vi "TEST-runner.vi"() -> ()   [LabVIEW 2016]
uses:
  Classes/Controllers/Motion/Copy of Motion Folder/Motion.lvclass
  Classes/Controllers/Camera/Copy of Controller Folder/Controller.lvclass
panel:
  in  "loop time":i32
  in  "START":bool
  in  "stop":bool
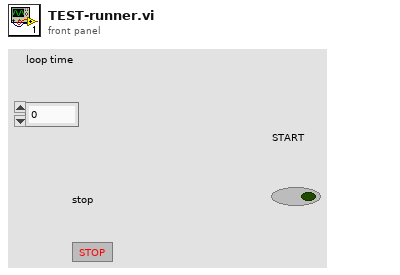
[diagram p1: front panel]
types:
  T1 = typedef "Controller.lvclass/Controllers.ctl" = cluster{"Copy of Motion.lvclass":refnum<class "Motion.lvclass">, "Copy of I-O.lvclass":refnum<class "I-O.lvclass">, "Copy of Dispenser.lvclass":refnum<class "Dispenser.lvclass">}
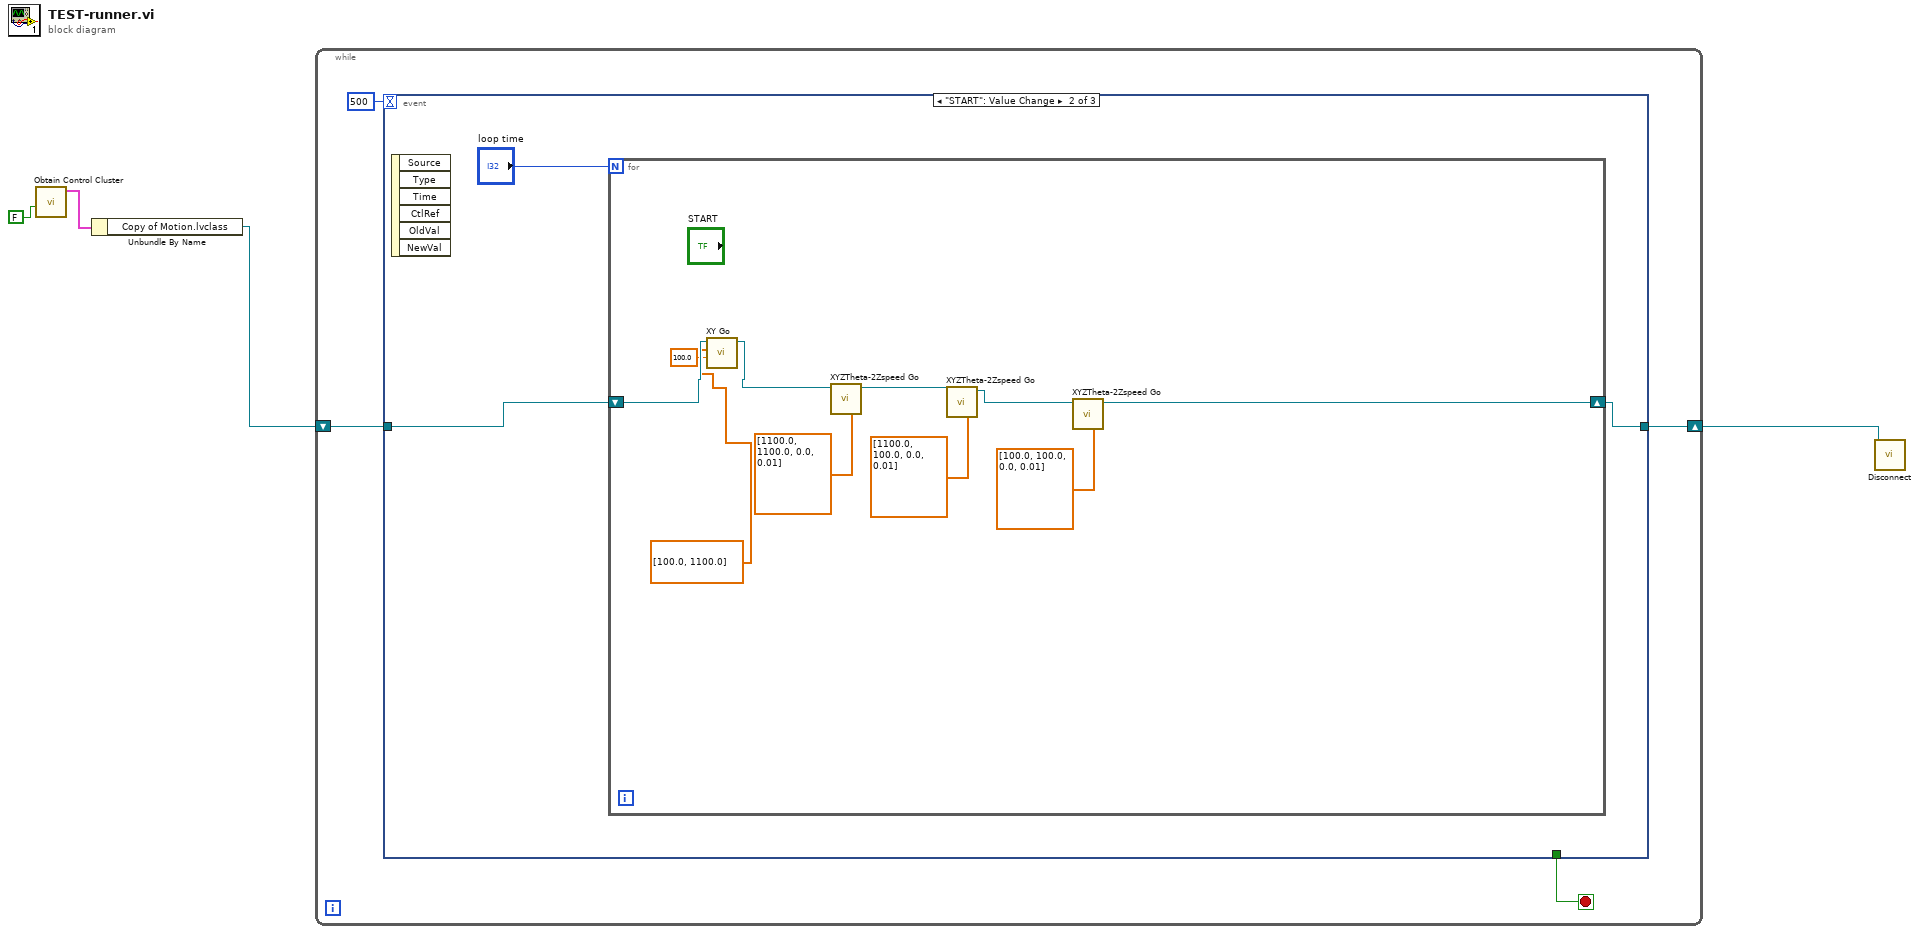
[diagram p0: block diagram]
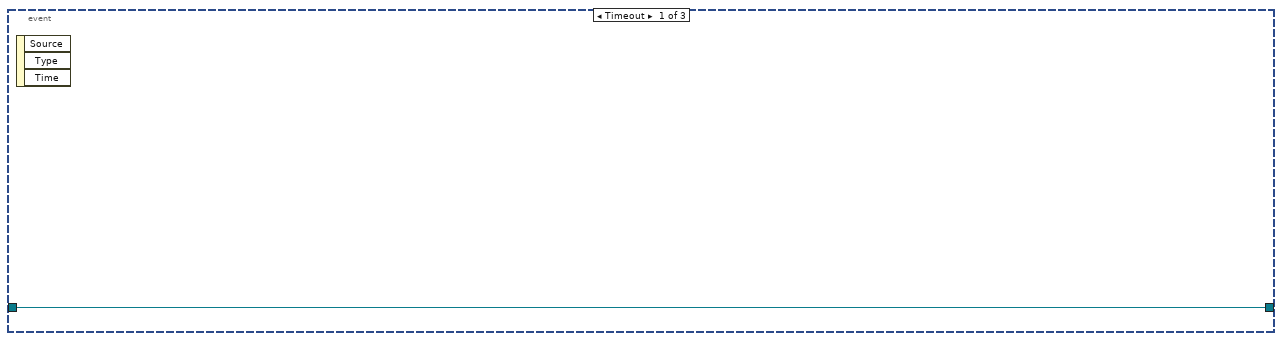
[diagram p2: hidden frame]
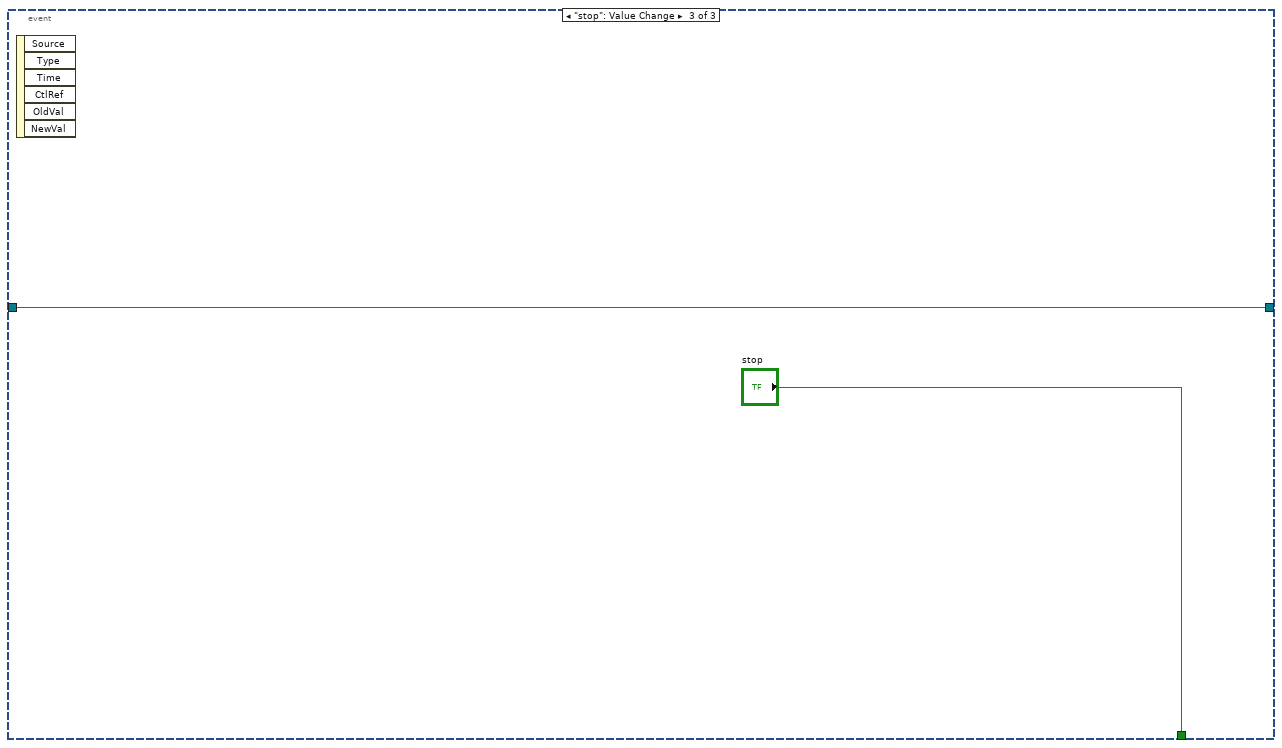
[diagram p3: hidden frame]
diagram:
  n1 = call "Obtain Control Cluster.vi"("I/O"=FALSE) -> ("Control Out"=w4:T1)  [unwired: 10 in]
  n2 = Unbundle By Name(w4) -> ("Copy of Motion.lvclass"=w2:refnum<class "Motion.lvclass">)
  n3 = while {
    shift-right: [w7] -> w1
    shift-left: w2 -> [w8]
    stop <- w5 stop-if-true
    n4 = event shown="[1] \"START\": Value Change" {
      selector: _ -> [_ _ _]
      dyn-events: _ -> [_ _ _]
      timeout: 500 -> [_ _ _]
      tunnel: w8 -> [w9 w11 w24]
      tunnel: [w9 w10 w24] -> w7
      tunnel: [_ _ "stop"] -> w5
      event Timeout {
        n5 = event-data() -> ()  [unwired: 1 in, 3 out]
      }
      event "START": Value Change {
        n6 = event-data() -> ()  [unwired: 1 in, 6 out]
        n7 = for {
          N: "loop time" -> [_]
          shift-right: [w17] -> w10
          shift-left: w11 -> [w16]
          n8 = call-dynamic "XY Go.vi"("Speed"=100.0, "XY"=dbl[] [100.0, 1100.0], "Motion in"=w16) -> ("Motion out"=w15:refnum<class "Motion.lvclass">)  [unwired: 7 in, 1 out]
          n9 = call "XYZTheta-2Zspeed Go.vi"("XYZTheta In"=dbl[] [1100.0, 1100.0, 0.0, 0.01] ("Parking position"), "Motion in"=w15) -> ("Motion out"=w20:refnum<class "Motion.lvclass">)  [unwired: 7 in, 2 out]
          n10 = call "XYZTheta-2Zspeed Go.vi"("XYZTheta In"=dbl[] [1100.0, 100.0, 0.0, 0.01] ("Parking position"), "Motion in"=w20) -> ("Motion out"=w18:refnum<class "Motion.lvclass">)  [unwired: 7 in, 2 out]
          n11 = call "XYZTheta-2Zspeed Go.vi"("XYZTheta In"=dbl[] [100.0, 100.0, 0.0, 0.01] ("Parking position"), "Motion in"=w18) -> ("Motion out"=w17:refnum<class "Motion.lvclass">)  [unwired: 7 in, 2 out]
        }
      }
      event "stop": Value Change {
        n12 = event-data() -> ()  [unwired: 1 in, 6 out]
      }
    }
  }
  n13 = call-dynamic "Disconnect.vi"("Controller in"=w1) -> ()  [unwired: 9 in, 1 out]
